vi "Read Supported Functions.vi"(8 "error in (no error)":errorcluster, 11 "Stanford Research in":refnum<class "Stanford Research.lvclass">) -> (0 "error out":errorcluster, 2 "Supported Functions":T1[](array[typedef])=[enum."Input"], 3 "Stanford Research out":refnum<class "Stanford Research.lvclass">)   [LabVIEW 2015, in "Stanford Research.lvclass"]
uses:
  Stanford Research.lvclass
  Mag Lab Hardware Function.ctl
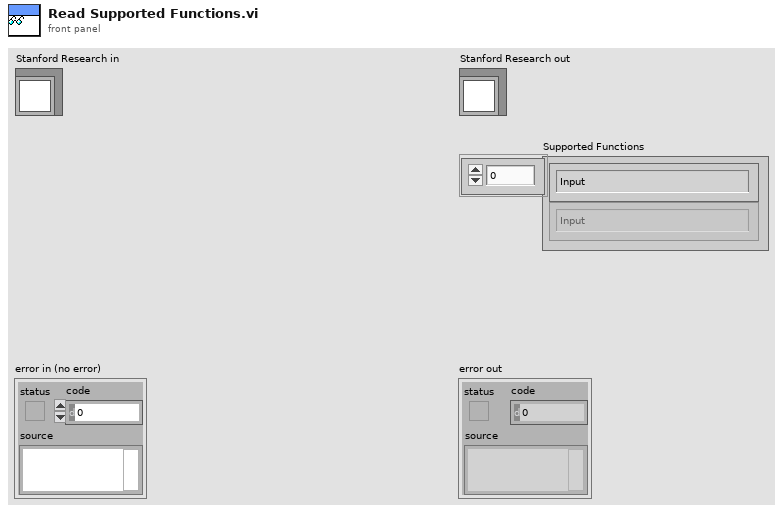
[diagram p1: front panel]
types:
  T1 = typedef "Mag Lab Hardware Function.ctl" = enum16{"Input", "Voltmeter", "Output", "Current source", "Digitizer", "Temperature controller"}
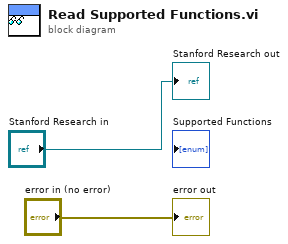
[diagram p0: block diagram]
diagram:
  "error out" <- "error in (no error)"
  "Stanford Research out" <- "Stanford Research in"
